vi "save_apollo_test_log.vi"(8 "error in (no error)":errorcluster, 11 "Test name":string) -> (0 "error out":errorcluster)   [LabVIEW 2010]
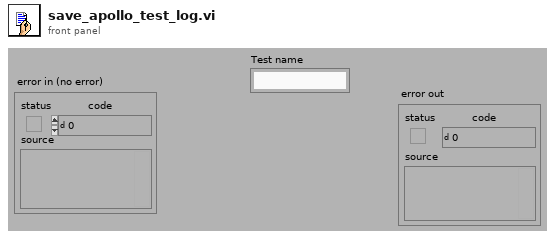
[diagram p1: front panel]
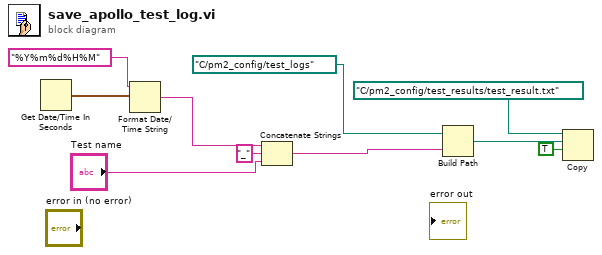
[diagram p0: block diagram]
diagram:
  n1 = Get Date/Time In Seconds() -> (seconds since 1Jan1904=w10:timestamp)
  n2 = Format Date/Time String(time format string (%c)="%Y%m%d%H%M", seconds (now)=w10) -> (date/time string=w8:string)  [unwired: 1 in]
  n3 = Concatenate Strings(w8, "_" ("string"), "Test name") -> (w7:string)
  n4 = Build Path(base path=path "C:/pm2_config/test_logs" ("file path (use dialog)"), name or relative path=w7) -> (appended path=w5:path)
  n5 = Copy(9:TRUE ("overwrite (F)"), 10:w5, 11:path "C:/pm2_config/test_results/test_result.txt" ("source path")) -> ()  [unwired: 2 in, 3 out]
